vi "calc_Z.vi"(0 "CO2A W":dbl format="%#_13g", 5 "CO2B W":dbl format="%#_13g", 9 "temp":dbl format="%#_13g", 11 "Chi CO2 A (ref)":dbl format="%#_13g") -> (8 "Z":dbl format="%#_13g")   [LabVIEW 2017, in "Licor-Steuerung.lvlib"]
uses:
  Licor-Steuerung.lvlib
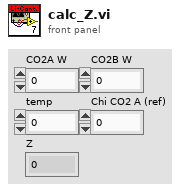
[diagram p1: front panel]
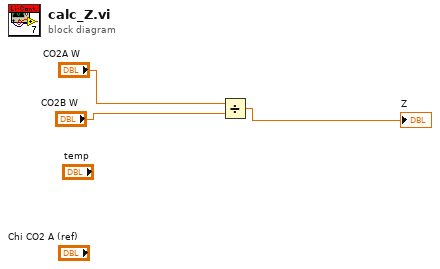
[diagram p0: block diagram]
diagram:
  n1 = Divide(x="CO2A W", y="CO2B W") -> (x/y=→"Z":dbl)
